vi "Element address end.vi"(8 "Last package unpacked":bool, 9 "Output Valid":bool, 10 "Element address final":u32, 11 "Elements read counter":u32) -> (1 "All elements read":bool, 3 "Next element address":u32)   [LabVIEW 2015]
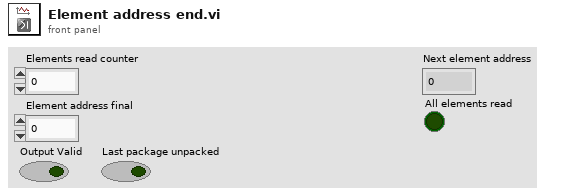
[diagram p1: front panel]
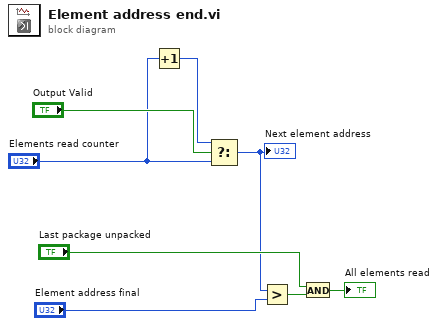
[diagram p0: block diagram]
diagram:
  n1 = Increment(x="Elements read counter") -> (x+1=w8:u32)
  n2 = Select(t=w8, s="Output Valid", f="Elements read counter") -> (s? t:f=w1:u32)
  "Next element address" <- w1
  n3 = Greater?(x=w1, y="Element address final") -> (0:w3:bool)
  n4 = And(x="Last package unpacked", y=w3) -> (x .and. y?=→"All elements read":bool)
